vi "Instance.vi"(10 "error in (no error)":errorcluster) -> (2 "error out":errorcluster, 3 "Platform Manager":refnum<class "PlatformPluginManager.lvclass">)   [LabVIEW 2020, in "PicoG-Core.lvlib" / "PlatformPluginManager.lvclass"]
uses:
  PlatformPluginManager.lvclass
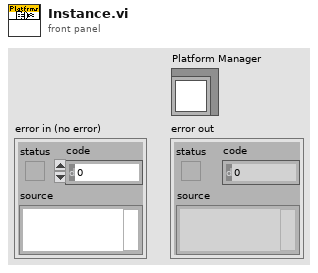
[diagram p1: front panel]
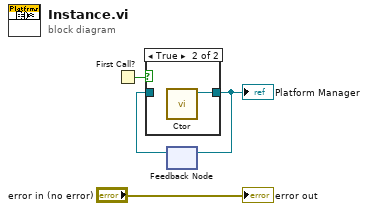
[diagram p0: block diagram]
diagram:
  n1 = First Call?() -> (First Call?: T/F=w3:bool)
  n2 = feedback #1() -> (w1:refnum<class "PlatformPluginManager.lvclass">)  [unwired: 1 in]
  n3 = case shown="True" w3 {
    tunnel: [w5 w6] -> w2
    tunnel: w1 -> [w5 _]
    frame False {
    }
    frame True {
      n4 = call "Ctor.vi"() -> ("TargetPluginManager out"=w6:refnum<class "PlatformPluginManager.lvclass">)  [unwired: 10 in, 1 out]
    }
  }
  "Platform Manager" <- w2
  n5 = feedback-in #1(w2) -> ()
  "error out" <- "error in (no error)"
